vi "Check refnum if its IA CD.vi"(8 "Error In":errorcluster, 11 "Refnum In":T1 format="%.0x") -> (0 "Error Out":errorcluster, 2 "Is Instrument Addon?":bool, 3 "Refnum Out":T1 format="%.0x")   [LabVIEW 2018, in "Instrument Addon Scripting API.lvlib"]
doc: "Verifies if the provided Refnum is an Instrument Addon Custom Device\n\nInput: \nRefnum In: represent the reference number which about to be compared agains the Instrument Addon GUID\n\nOutput: \nRefnum Out: represents the reference number provided as input\nIs Instrument Addon?: boolean value which indicates if the provided refnum references an Instrument Addon Custom Device"
uses:
  Instrument Addon Scripting API.lvlib
  <vilib>/NI Veristand/Custom Device API/Custom Device Item Ref.ctl
  Addon/Addon Shared/SubVIs/Constants.vi
  <vilib>/Utility/error.llb/Error Cluster From Error Code.vi
  <vilib>/ErrorRing/Error Ring.xnode
  <vilib>/NI/NI VeriStand Advanced SysDef API/SysDef API/Advanced System Definition.lvlib
  Addon/Addon Shared/Instrument Addon Shared.lvlib
  <vilib>/NI Veristand/Custom Device API/Custom Device API.lvlib
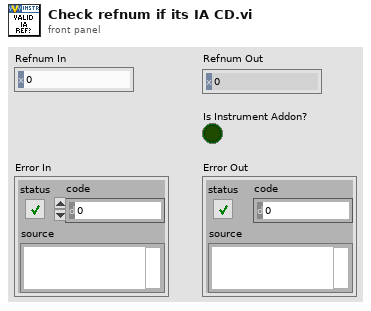
[diagram p1: front panel]
types:
  T1 = typedef "Custom Device API.lvlib/Custom Device Item Ref.ctl" = u64
  T2 = typedef "Advanced System Definition.lvlib/TreeItem.Info.ctl" = cluster{"Name":string, "Description":string, "GUID":string, "Is Channel":bool, "Channel":T3, "Is Waveform":bool, "Waveform":T5}
  T3 = typedef "Custom Device API.lvlib/Custom Device Channel.ctl" = cluster{"Type":T4, "Units":string, "Default Value":dbl, "Faultable":bool, "Scalable":bool}
  T4 = typedef "Custom Device API.lvlib/Custom Device Channel Type.ctl" = enum16{"Input", "Output"}
  T5 = typedef "Custom Device API.lvlib/Custom Device Waveform.ctl" = cluster{"Data Type":T6, "Units":string}
  T6 = typedef "Custom Device API.lvlib/Custom Device Waveform DataType.ctl" = enum16{"Double", "Complex Double"}
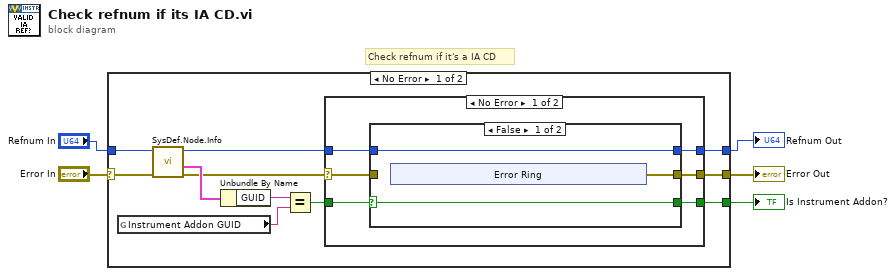
[diagram p0: block diagram]
diagram:
  # "Check refnum if it's a IA CD"
  n1 = case shown="No Error" "Error In" {
    selector: "Error In" -> [w12 w37]
    tunnel: [w11 w37] -> w5
    tunnel: [w9 w38] -> w1
    tunnel: "Refnum In" -> [w13 w38]
    tunnel: [w8 _] -> w3
    frame No Error {
      n2 = global read "Constants.vi" "Instrument Addon GUID"() -> (w16:string)
      n3 = call <vilib>:"SysDef.Node.Info.vi"("error in (no error)"=w12, "nodeID"=w13) -> ("error out"=w7:errorcluster, "Item Info"=w14:T2, "nodeID out"=w10:u64)  [unwired: 6 in, 1 out]
      n4 = Unbundle By Name(w14) -> ("GUID"=w15:string)
      n5 = Equal?(x=w15, y=w16) -> (x = y?=w6:bool)
      n6 = case shown="No Error" w7 {
        selector: w7 -> [w18 w36]
        tunnel: [w22 w36] -> w11
        tunnel: w10 -> [w21 w35]
        tunnel: [w20 w35] -> w9
        tunnel: [w19 w34] -> w8
        tunnel: w6 -> [w17 w34]
        frame No Error {
          n7 = case shown="False" w17 {
            selector: w17 -> [w23 w32]
            tunnel: [w24 w31] -> w22
            tunnel: w21 -> [w25 w33]
            tunnel: [w25 w33] -> w20
            tunnel: [w23 w32] -> w19
            tunnel: w18 -> [_ w31]
            frame False {
              n8 = xnode "Error Ring"() -> ("error out"=w24:errorcluster)
            }
            frame True {
            }
          }
        }
        frame Error {
        }
      }
    }
    frame Error {
    }
  }
  "Error Out" <- w5
  "Is Instrument Addon?" <- w3
  "Refnum Out" <- w1
